vi "taskTrial_multiPlatform.vi"(0 "Start \nplatform":i32, 1 "Rat ID":string, 3 "difficulty":dbl, 5 "Goal \nplatform":i32, 7 "Max number of platforms to \npick":i32=2, 9 "previousChoices":i32[][](array[numeric]), 11 "error in (no error)":errorcluster, 12 "up or down":string, 14 "mazeDirection":string) -> (4 "choicesCurrent":i32[][](array[numeric]), 10 "previousChoices updated":i32[][](array[numeric]), 15 "error out":errorcluster)   [LabVIEW 2017]
panel:
  out "array w/ subset deleted":i32[](array[numeric])
  out "appended array":i32[](array[numeric])
  out "new\nplatform":i32
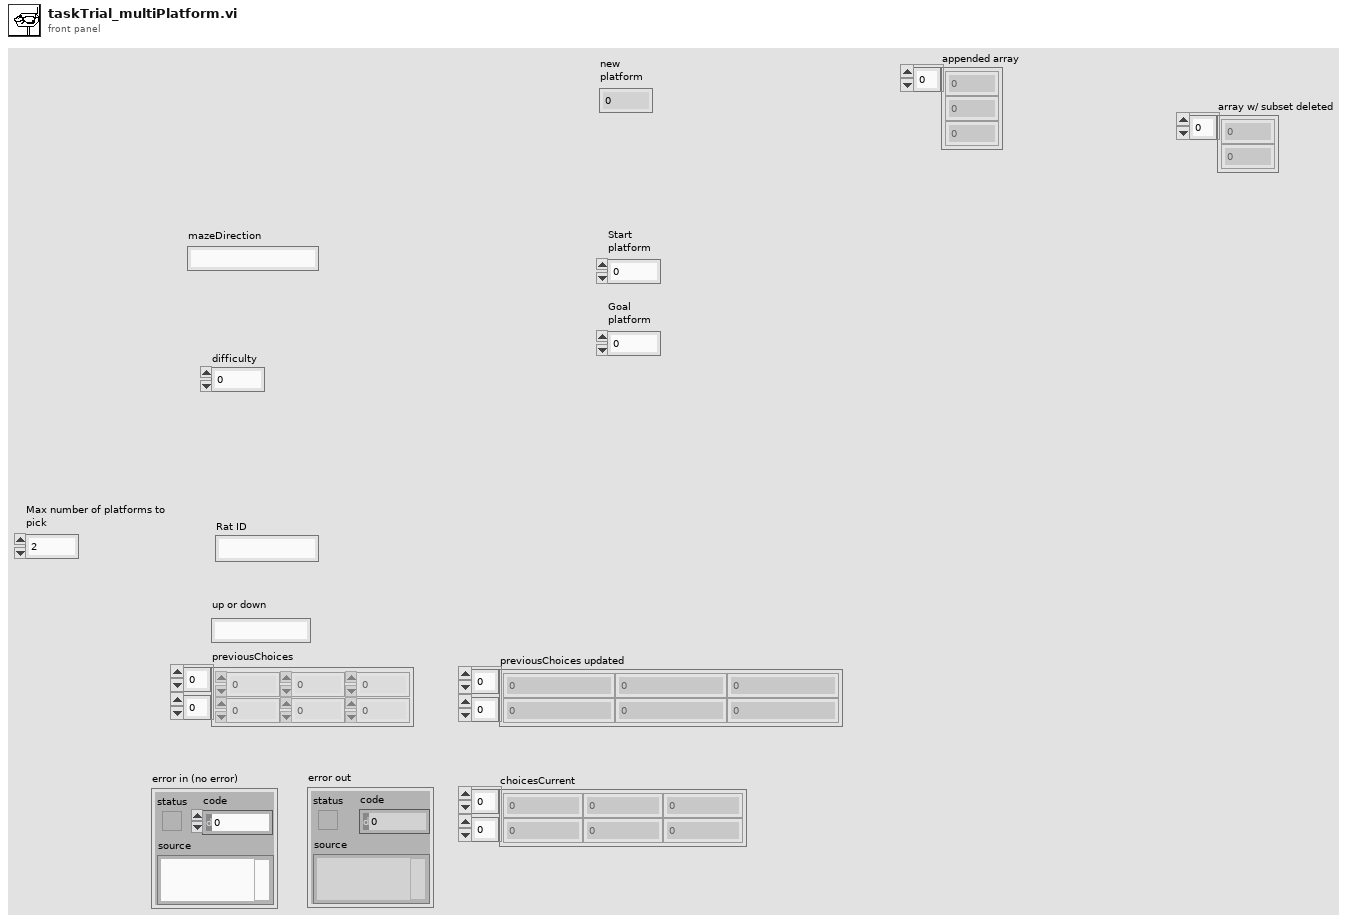
[diagram p1: front panel]
types:
  T1 = enum16{"open", "replace", "create", "open or create", "replace or create", "replace or create with confirmation"}
  T2 = enum16{"big-endian, network order", "native, host order", "little-endian"}
  T3 = cluster{"normal time":dbl, "high res \nrelative time":dbl, "high res \nrelative time":dbl, "Numeric":dbl, "Numeric":dbl, "Numeric":dbl, "vector length":dbl, "vector length":dbl, "vector length":dbl, "vector \nangle":dbl, "vector \nangle":dbl, "vector \nangle":dbl, dbl}
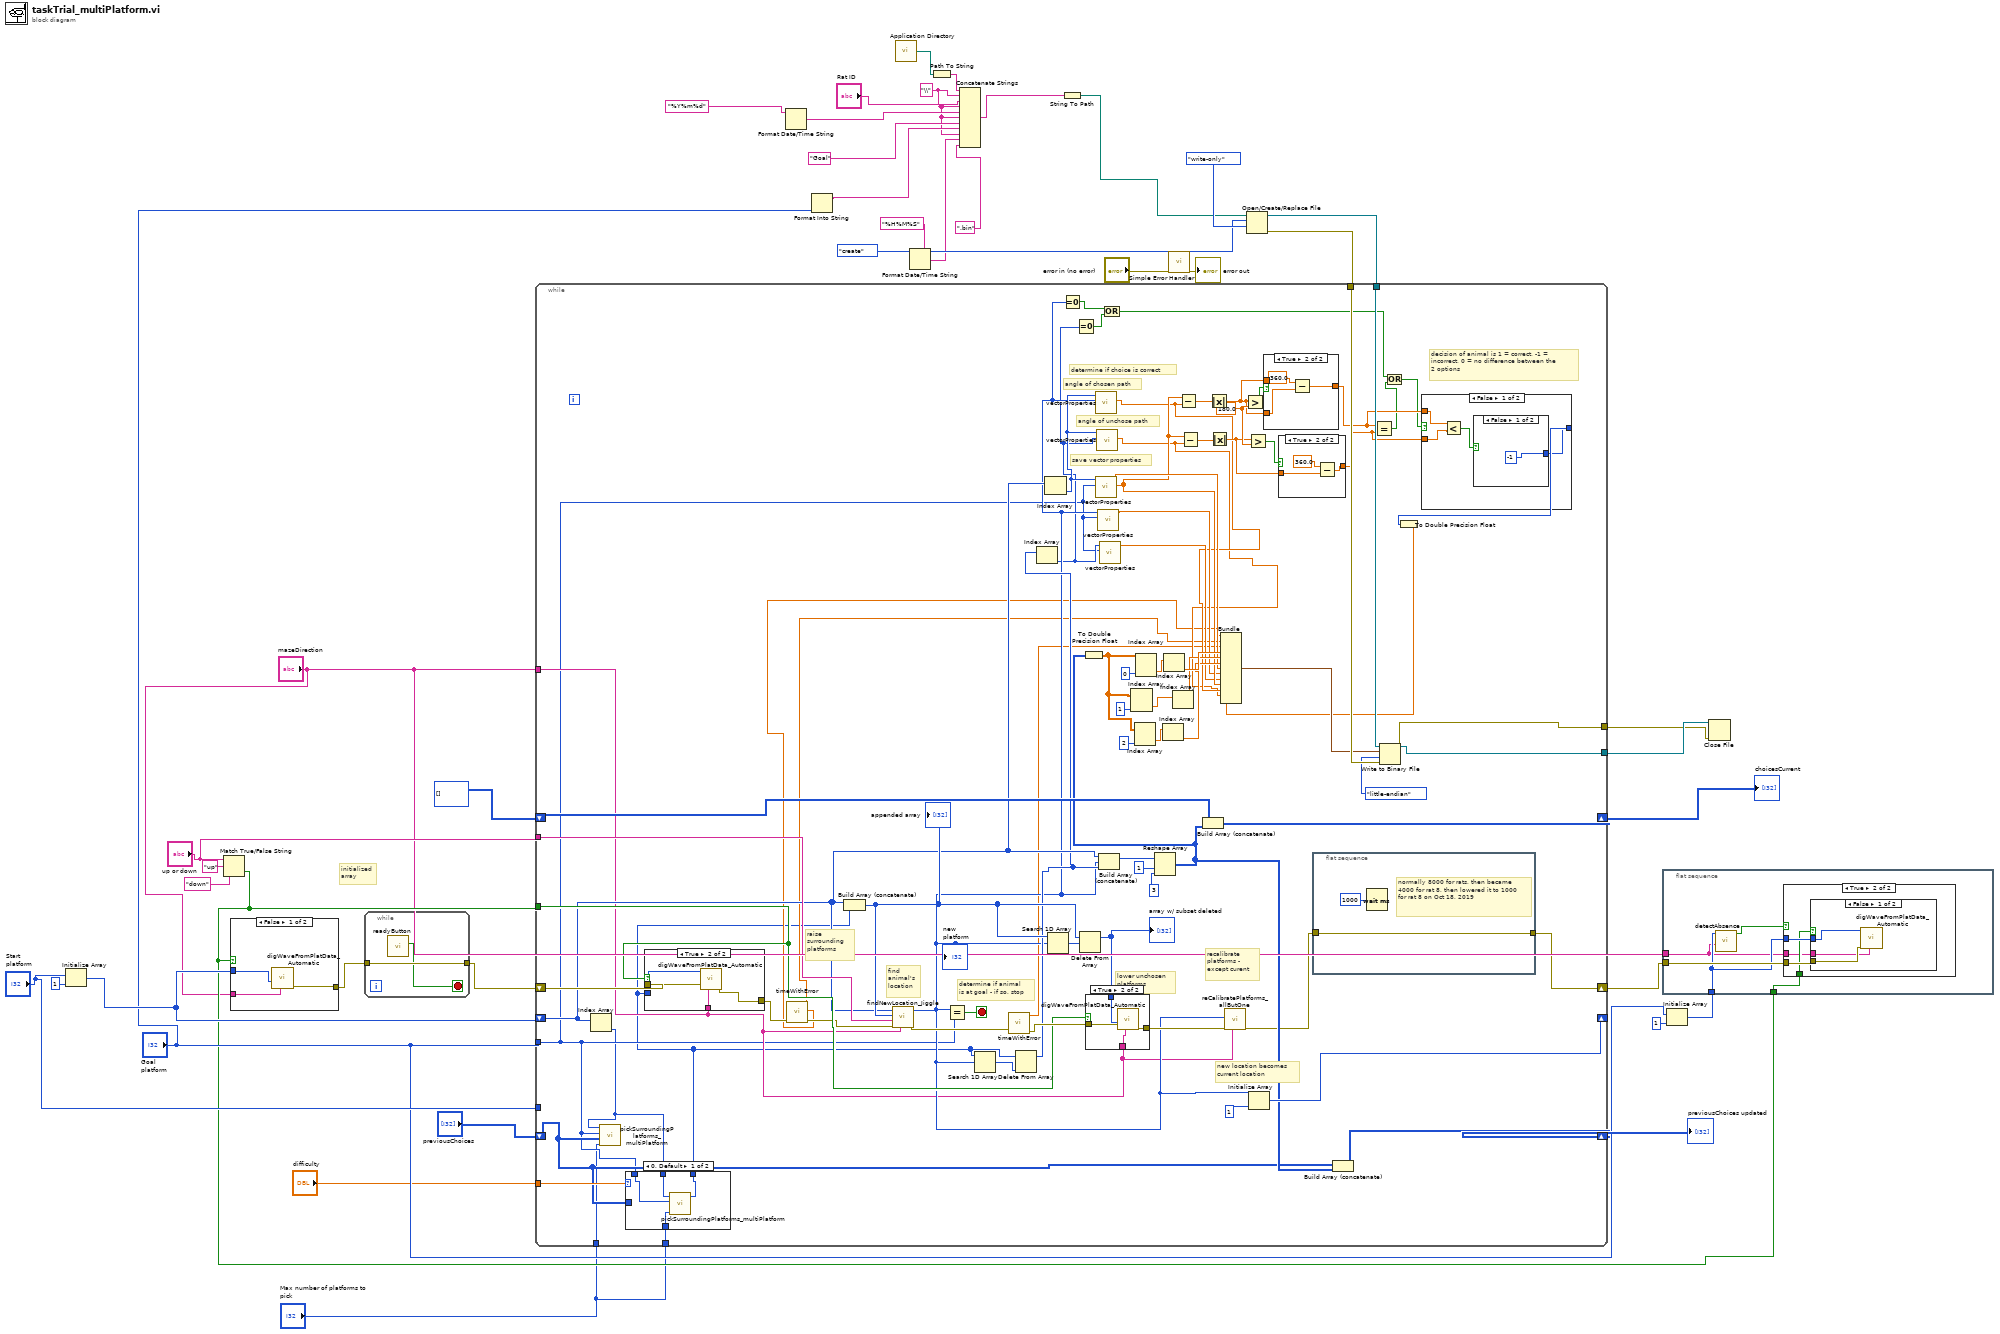
[diagram p0: block diagram]
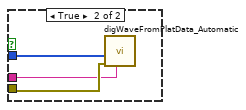
[diagram p3: hidden frame]
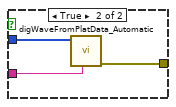
[diagram p4: hidden frame]
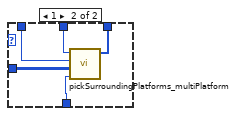
[diagram p5: hidden frame]
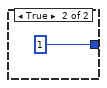
[diagram p6: hidden frame]
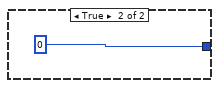
[diagram p7: hidden frame]
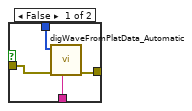
[diagram p10: hidden frame]
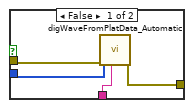
[diagram p11: hidden frame]
diagram:
  w19 = "\\" ("string")
  # "initialized\narray"
  n1 = Initialize Array("Start \nplatform", 1 ("dimension size")) -> (w35:i32[])
  n2 = Match True/False String(2:"down" ("false string"), 3:"up" ("true string"), 4:"up or down") -> (0:w4:bool)  [unwired: 1 out]
  n3 = case shown="False" w4 {
    tunnel: [w44 w47] -> w10
    tunnel: w35 -> [w43 w46]
    tunnel: "mazeDirection" -> [w42 w45]
    frame False {
      n4 = call "digWaveFromPlatData_Automatic.vi"("mazeDirection"=w42, "Platforms\nto lower"=w43) -> ("error out"=w44:errorcluster)  [unwired: 9 in]
    }
    frame True {
      n5 = call "digWaveFromPlatData_Automatic.vi"("mazeDirection"=w45, "Platforms\nto raise"=w46) -> ("error out"=w47:errorcluster)  [unwired: 9 in]
    }
  }
  n6 = while {
    tunnel: w10 -> [w49]
    tunnel: [w49] -> w9
    stop <- w48 stop-if-true
    n7 = call "readyButton.vi"() -> ("Ready? 2"=w48:bool)  [unwired: 9 in]
  }
  n8 = Format Date/Time String(time format string (%c)="%Y%m%d" ("time string")) -> (date/time string=w21:string)  [unwired: 2 in]
  n9 = Format Into String("Goal \nplatform") -> (resulting string=w22:string)  [unwired: 3 in, 1 out]
  n10 = call <vilib>:"Application Directory.vi"() -> ("Application Directory"=w24:path)
  n11 = Format Date/Time String(time format string (%c)="%H%M%S" ("time string")) -> (date/time string=w17:string)  [unwired: 2 in]
  n12 = Path To String(path=w24) -> (string=w27:string)
  n13 = Concatenate Strings(w27, w19, "Rat ID", w19, w21, w19, "Goal" ("string"), w22, w19, w17, ".bin") -> (w15:string)
  n14 = String To Path(string=w15) -> (path=w23:path)
  n15 = call <vilib>:"Simple Error Handler.vi"("error in (no error)"="error in (no error)") -> ("error out"=→"error out":errorcluster)  [unwired: 4 in, 4 out]
  n16 = Open/Create/Replace File(file path (use dialog)=w23, operation (0:open)=T1."create", access (0:read/write)=enum16{"read/write", "read-only", "write-only"}."write-only") -> (refnum out=w31:refnum<file>, error out=w30:errorcluster)  [unwired: 3 in, 1 out]
  n17 = while {
    tunnel: "Goal \nplatform" -> [w54]
    shift-right: [w90] -> w8
    shift-left: w9 -> [w122]
    shift-right: [w113] -> w40
    shift-left: i32[][] [] -> [w121]
    shift-right: [w117] -> w39
    shift-left: "previousChoices" -> [w55]
    shift-right: [w116] -> _
    shift-left: w35 -> [w89]
    tunnel: w31 -> [w112]
    tunnel: w30 -> [w111]
    tunnel: [w109] -> w29
    tunnel: [w108] -> w28
    tunnel: w4 -> [w92]
    tunnel: "up or down" -> [w93]
    tunnel: "Start \nplatform" -> [_]
    tunnel: "mazeDirection" -> [w57]
    tunnel: "difficulty" -> [w56]
    tunnel: "Max number of platforms to \npick" -> [w51]
    tunnel: "Max number of platforms to \npick" -> [w50]
    stop <- w125 stop-if-true
    w84 = 180.0 ("y")
    # "decision of animal is 1 = correct, -1 = \nincorrect, 0 = no difference between the \n2 options"
    # "angle of unchose path"
    # "angle of chosen path"
    # "save vector properties"
    # "determine if choice is correct"
    # "determine if animal \nis at goal - if so, stop"
    # "new location becomes\ncurrent location"
    # "recalibrate \nplatforms - \nexcept curent"
    # "lower unchosen\nplatforms"
    # "find \nanimal's \nlocation"
    # "raise \nsurrounding \nplatforms"
    n18 = Index Array(array=w89) -> (element=w53:i32)  [unwired: 1 in]
    n19 = call "pickSurroundingPlatforms_multiPlatform.vi"("Max number of platforms to \npick"=w51, "previousChoices"=w55, "Goal \nplatform"=w54, "Start platform"=w53) -> ()  [unwired: 7 in, 1 out]
    n20 = case shown="0, Default" w56 {
      tunnel: w55 -> [_ w136]
      tunnel: w54 -> [w131 w135]
      tunnel: w53 -> [w129 w134]
      tunnel: [w130 w133] -> w52
      tunnel: w50 -> [w128 w132]
      frame 0, Default {
        n21 = call "pickSurroundingPlatforms_multiPlatform.vi"("Max number of platforms to \npick"=w128, "Goal \nplatform"=w131, "Start platform"=w129) -> ("platform choices"=w130:i32[])  [unwired: 8 in]
      }
      frame 1 {
        n22 = call "pickSurroundingPlatforms_multiPlatform.vi"("Max number of platforms to \npick"=w132, "previousChoices"=w136, "Goal \nplatform"=w135, "Start platform"=w134) -> ("platform choices"=w133:i32[])  [unwired: 7 in]
      }
    }
    n23 = case shown="True" w92 {
      tunnel: w122 -> [w164 w169]
      tunnel: [w163 w168] -> w62
      tunnel: w52 -> [w165 w167]
      tunnel: w57 -> [w162 w166]
      frame False {
        n24 = call "digWaveFromPlatData_Automatic.vi"("mazeDirection"=w162, "error in (no error)"=w164, "Platforms\nto lower"=w165) -> ("error out"=w163:errorcluster)  [unwired: 8 in]
      }
      frame True {
        n25 = call "digWaveFromPlatData_Automatic.vi"("mazeDirection"=w166, "error in (no error)"=w169, "Platforms\nto raise"=w167) -> ("error out"=w168:errorcluster)  [unwired: 8 in]
      }
    }
    n26 = call "timeWithError.vi"("error in (no error)"=w62) -> ("high res \nrelative time"=w60:dbl, "normal time"=w59:dbl, "error out"=w61:errorcluster)  [unwired: 7 in]
    n27 = Build Array (concatenate)(w89, w52) -> (w115:i32[])
    "appended array" <- w115
    n28 = call "findNewLocation_Jiggle.vi"("mazeDirection"=w57, "error in (no error)"=w61, "up or down"=w93, "possible \nlocations"=w115, "start \nlocation"=w89) -> ("error out"=w94:errorcluster, "new\nplatform"=w75:i32)  [unwired: 5 in]
    "new\nplatform" <- w75
    n29 = Equal?(x=w75, y=w54) -> (x = y?=w125:bool)
    n30 = Search 1D Array(1D array=w52, element=w75) -> (index of element=w114:i32)  [unwired: 1 in]
    n31 = call "timeWithError.vi"("error in (no error)"=w94) -> ("high res \nrelative time"=w58:dbl, "error out"=w95:errorcluster)  [unwired: 7 in, 1 out]
    n32 = Delete From Array(array=w52, index=w114) -> (array with subset deleted=w88:i32[])  [unwired: 1 in, 1 out]
    n33 = Index Array(array=w88) -> (element=w74:i32)  [unwired: 1 in]
    n34 = Index Array(array=w89) -> (element=w87:i32)  [unwired: 1 in]
    n35 = Search 1D Array(1D array=w115, element=w75) -> (index of element=w127:i32)  [unwired: 1 in]
    n36 = Equal To 0?(x=w75) -> (x = 0?=w72:bool)
    n37 = Equal To 0?(x=w74) -> (x = 0?=w73:bool)
    n38 = Delete From Array(array=w115, index=w127) -> (array with subset deleted=w126:i32[])  [unwired: 1 in, 1 out]
    "array w/ subset deleted" <- w126
    n39 = case shown="True" w92 {
      tunnel: w126 -> [w157 w161]
      tunnel: [w155 w160] -> w123
      tunnel: w95 -> [w156 w159]
      tunnel: w57 -> [w154 w158]
      frame False {
        n40 = call "digWaveFromPlatData_Automatic.vi"("mazeDirection"=w154, "error in (no error)"=w156, "Platforms\nto raise"=w157) -> ("error out"=w155:errorcluster)  [unwired: 8 in]
      }
      frame True {
        n41 = call "digWaveFromPlatData_Automatic.vi"("mazeDirection"=w158, "error in (no error)"=w159, "Platforms\nto lower"=w161) -> ("error out"=w160:errorcluster)  [unwired: 8 in]
      }
    }
    n42 = call "vectorProperties.vi"("Goal \nplatform"=w75, "Start \nplatform"=w87) -> ("vector \nangle"=w64:dbl)  [unwired: 8 in, 1 out]
    n43 = call "vectorProperties.vi"("Goal \nplatform"=w54, "Start \nplatform"=w87) -> ("vector \nangle"=w67:dbl, "vector length"=w68:dbl)  [unwired: 8 in]
    n44 = call "vectorProperties.vi"("Goal \nplatform"=w74, "Start \nplatform"=w87) -> ("vector \nangle"=w63:dbl)  [unwired: 8 in, 1 out]
    n45 = call "vectorProperties.vi"("Goal \nplatform"=w54, "Start \nplatform"=w75) -> ("vector length"=w66:dbl)  [unwired: 8 in, 1 out]
    n46 = Build Array (concatenate)(w89, w75, w88) -> (w118:i32[])
    n47 = call "vectorProperties.vi"("Goal \nplatform"=w54, "Start \nplatform"=w74) -> ("vector length"=w65:dbl)  [unwired: 8 in, 1 out]
    n48 = Or(x=w72, y=w73) -> (x .or. y?=w71:bool)
    n49 = Reshape Array(w118, 1 ("dimension size"), 3 ("dimension size")) -> (w107:i32[][])
    n50 = To Double Precision Float(number=w107) -> (double precision float=w101:dbl[][])
    n51 = Index Array(array=w101, index (col)=1 ("disabled index (col)")) -> (element=w102:dbl[])  [unwired: 1 in]
    n52 = Index Array(array=w101, index (col)=2 ("disabled index (col)")) -> (element=w99:dbl[])  [unwired: 1 in]
    n53 = Index Array(array=w101, index (col)=0 ("disabled index (col)")) -> (element=w105:dbl[])  [unwired: 1 in]
    n54 = Index Array(array=w99) -> (element=w97:dbl)  [unwired: 1 in]
    n55 = Index Array(array=w105) -> (element=w104:dbl)  [unwired: 1 in]
    n56 = Index Array(array=w102) -> (element=w98:dbl)  [unwired: 1 in]
    n57 = Subtract(x=w67, y=w64) -> (x-y=w86:dbl)
    n58 = Subtract(x=w67, y=w63) -> (x-y=w85:dbl)
    n59 = Build Array (concatenate)(w121, w107) -> (w113:i32[][])
    n60 = Absolute Value(x=w86) -> (abs(x)=w82:dbl)
    n61 = Absolute Value(x=w85) -> (abs(x)=w80:dbl)
    n62 = call "reCalibratePlatforms_allButOne.vi"("mazeDirection"=w57, "error in (no error)"=w123, "Current location"=w75) -> ("error out"=w91:errorcluster)  [unwired: 8 in]
    n63 = Greater?(x=w82, y=w84) -> (0:w83:bool)
    n64 = Greater?(x=w80, y=w84) -> (0:w81:bool)
    n65 = Initialize Array(w75, 1 ("dimension size")) -> (w116:i32[])
    n66 = case shown="True" w83 {
      tunnel: w82 -> [_ w150]
      tunnel: [w148 w149] -> w79
      tunnel: w82 -> [w148 _]
      frame False {
      }
      frame True {
        n67 = Subtract(x=360.0, y=w150) -> (x-y=w149:dbl)
      }
    }
    n68 = case shown="True" w81 {
      tunnel: w80 -> [w144 w146]
      tunnel: [w144 w145] -> w78
      frame False {
      }
      frame True {
        n69 = Subtract(x=360.0, y=w146) -> (x-y=w145:dbl)
      }
    }
    n70 = flat-sequence {
      tunnel: w91 -> [w153]
      tunnel: [w153] -> w90
      frame #0 {
        # "normally 8000 for rats, then became 4000 for rat 8, then lowered it to 1000 for rat 8 on Oct 18, 2019"
        n71 = Wait (ms)(milliseconds to wait=u32 1000) -> ()  [unwired: 1 out]
      }
    }
    n72 = Build Array (concatenate)(w55, w107) -> (w117:i32[][])
    n73 = Equal?(x=w79, y=w78) -> (x = y?=w70:bool)
    n74 = Or(x=w71, y=w70) -> (x .or. y?=w69:bool)
    n75 = case shown="False" w69 {
      tunnel: [w137 0] -> w77
      tunnel: w79 -> [w140 _]
      tunnel: w78 -> [w139 _]
      frame False {
        n76 = Less?(x=w140, y=w139) -> (x < y?=w138:bool)
        n77 = case shown="False" w138 {
          tunnel: [-1 1] -> w137
          frame False {
          }
          frame True {
          }
        }
      }
      frame True {
      }
    }
    n78 = To Double Precision Float(number=w77) -> (double precision float=w76:dbl)
    n79 = Bundle("normal time"=w59, "high res \nrelative time"=w60, "high res \nrelative time"=w58, "Numeric"=w104, "Numeric"=w98, "Numeric"=w97, "vector length"=w68, "vector length"=w66, "vector length"=w65, "vector \nangle"=w67, "vector \nangle"=w64, "vector \nangle"=w63, w76) -> (w96:T3)  [unwired: 1 in]
    n80 = Write to Binary File(file (use dialog)=w112, data=w96, error in=w111, 9:T2."little-endian" ("byte order (0:big-endian, network order)")) -> (refnum out=w109:refnum<file>, error out=w108:errorcluster)  [unwired: 2 in, 1 out]
  }
  "choicesCurrent" <- w40
  "previousChoices updated" <- w39
  n81 = flat-sequence {
    tunnel: w8 -> [w174]
    tunnel: w5 -> [w173]
    tunnel: w4 -> [w171]
    tunnel: "mazeDirection" -> [w170]
    frame #0 {
      n82 = call "detectAbsence.vi"("mazeDirection"=w170, "platforms"=w173) -> ("Boolean"=w172:bool)  [unwired: 9 in]
      n83 = case shown="True" w172 {
        tunnel: w174 -> [_ w178]
        tunnel: w173 -> [_ w177]
        tunnel: w171 -> [_ w176]
        tunnel: w170 -> [_ w175]
        frame False {
        }
        frame True {
          n84 = case shown="False" w176 {
            tunnel: w178 -> [w180 w184]
            tunnel: w177 -> [w181 w183]
            tunnel: w175 -> [w179 w182]
            frame False {
              n85 = call "digWaveFromPlatData_Automatic.vi"("mazeDirection"=w179, "error in (no error)"=w180, "Platforms\nto raise"=w181) -> ()  [unwired: 8 in, 1 out]
            }
            frame True {
              n86 = call "digWaveFromPlatData_Automatic.vi"("mazeDirection"=w182, "error in (no error)"=w184, "Platforms\nto lower"=w183) -> ()  [unwired: 8 in, 1 out]
            }
          }
        }
      }
    }
  }
  n87 = Initialize Array("Goal \nplatform", 1 ("dimension size")) -> (w5:i32[])
  n88 = Close File(refnum=w29, error in=w28) -> ()  [unwired: 2 out]
